vi "QMH_Create_UI_Queue.vi"(8 "error in (no error)":errorcluster caption="entrée d'erreur (pas d'erreur)") -> (0 "error out":errorcluster caption="sortie d'erreur", 3 "UI Queue":refnum<queue>)   [LabVIEW 2015]
uses:
  controls/QMH_UI_Message.ctl
  controls/QMH_UI_Command.ctl
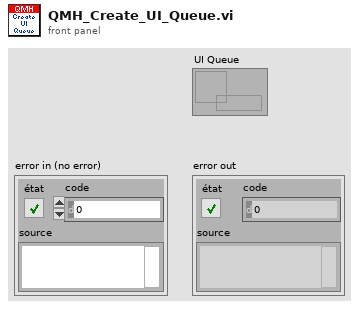
[diagram p1: front panel]
types:
  T1 = typedef "QMH_UI_Command.ctl" = enum16{"Initialize", "UI Load", "UI Save", "UI Change Experiment", "UI Change Voltages", "UI Change Sequence", "UI Change Expert", "Ready to Start", "UI Start", "UI Stop", "UI Exit", "Update Report", "Update ICR Report"}
  T2 = typedef "QMH_UI_Message.ctl" = cluster{"Command":T1, "Data":variant}
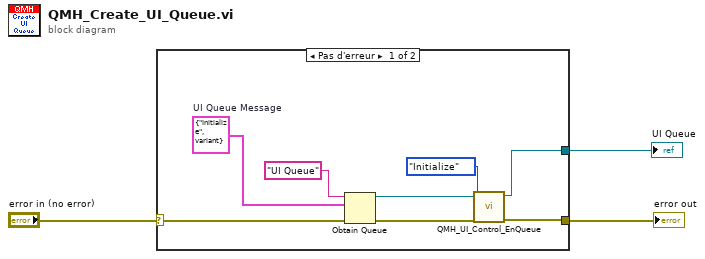
[diagram p0: block diagram]
diagram:
  n1 = case shown="Pas d'erreur" "error in (no error)" {
    selector: "error in (no error)" -> [w10 w12]
    tunnel: [w7 w12] -> w2
    tunnel: [w5 _] -> w1
    frame No Error {
      w9 = T2 {"Command"=enum."Initialize", "Data"=variant}  # UI Queue Message
      n2 = Obtain Queue(name (unnamed)="UI Queue" ("nom (aucun)"), element data type=w9, error in (no error)=w10) -> (queue out=w6:refnum<queue>, error out=w8:errorcluster)  [unwired: 2 in, 1 out]
      n3 = call "QMH_UI_Control_EnQueue.vi"("error in (no error)"=w8, "Command"=QMH_UI_Command."Initialize", "UI Queue"=w6) -> ("error out"=w7:errorcluster, "UI Queue"=w5:refnum<queue>)  [unwired: 7 in]
    }
    frame Error {
    }
  }
  "UI Queue" <- w1
  "error out" <- w2
